vi "FTW-TransferClient-Upload.vi"(0 "Transfer Client":refnum<k24>, 5 "Remote URI":string, 7 "Data":string, 11 "error in":errorcluster) -> (4 "Transfer Client out":refnum<k24>, 6 "URI":string, 8 "Response":string, 10 "Elapsed Time":dbl format="%.4psec", 15 "error out":errorcluster)   [LabVIEW 2014]
panel:
  # "Inputs"
  # "Outputs"
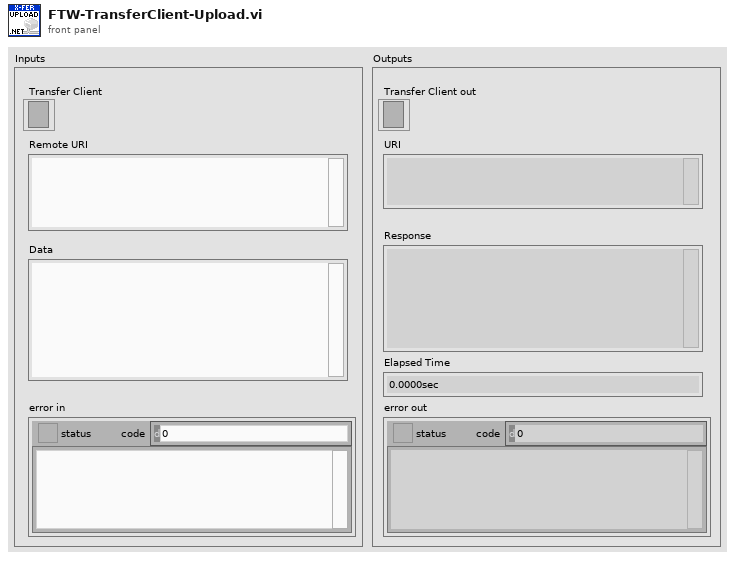
[diagram p1: front panel]
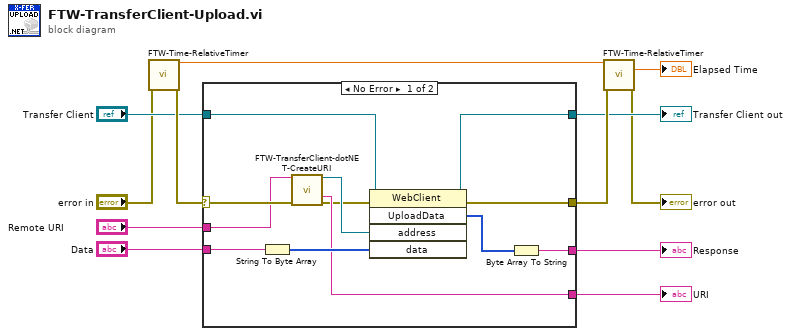
[diagram p0: block diagram]
diagram:
  n1 = call "FTW-Time-RelativeTimer.vi"("error in"="error in") -> ("Current Timer Value"=w10:dbl, "error out"=w12:errorcluster)  [unwired: 12 in, 1 out]
  n2 = case shown="No Error" w12 {
    selector: w12 -> [w16 w25]
    tunnel: "Transfer Client" -> [w14 w26]
    tunnel: [w24 _] -> w7
    tunnel: [w23 w25] -> w11
    tunnel: [w13 w26] -> w8
    tunnel: [w18 _] -> w6
    tunnel: "Data" -> [w21 _]
    tunnel: "Remote URI" -> [w15 _]
    frame No Error {
      n3 = String To Byte Array(string=w21) -> (unsigned byte array=w20:u8[])
      n4 = call "FTW-TransferClient-dotNET-CreateURI.vi"("URI"=w15, "error in"=w16) -> ("URI ref"=w19:refnum<k24>, "AbsoluteURI"=w18:string, "error out"=w17:errorcluster)  [unwired: 8 in, 3 out]
      n5 = invoke class="WebClient" method="UploadData"(reference=w14, error in=w17, "address"=w19, "data"=w20) -> (reference out=w13:refnum<k24>, error out=w23:errorcluster, "UploadData"=w22:u8[])  [unwired: 1 in, 2 out]
      n6 = Byte Array To String(unsigned byte array=w22) -> (string=w24:string)
    }
    frame Error {
    }
  }
  "Transfer Client out" <- w8
  "URI" <- w6
  "Response" <- w7
  n7 = call "FTW-Time-RelativeTimer.vi"("Previous Timer Value"=w10, "error in"=w11) -> ("Elapsed Time"=→"Elapsed Time":dbl, "error out"=→"error out":errorcluster)  [unwired: 11 in, 1 out]
